vi "CRYGetPaneArea.vi"(11 "vi reference":refnum<vi>) -> (3 "Content Area Rect":T1)   [LabVIEW 2013]
uses:
  <vilib>/Utility/miscctls.llb/LVRectTypeDef.ctl
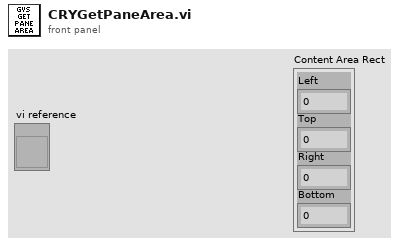
[diagram p1: front panel]
types:
  T1 = typedef "LVRectTypeDef.ctl" = cluster{"Left":i16, "Top":i16, "Right":i16, "Bottom":i16}
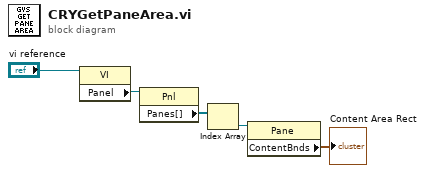
[diagram p0: block diagram]
diagram:
  n1 = property class="VI"(reference="vi reference") -> ("Panel"=w5:refnum<vi>)  [unwired: 1 in, 2 out]
  n2 = property class="Pnl"(reference=w5) -> ("Panes[]"=w4:refnum<vi>[])  [unwired: 1 in, 2 out]
  n3 = Index Array(array=w4) -> (element=w3:refnum<vi>)  [unwired: 1 in]
  n4 = property class="Pane"(reference=w3) -> ("ContentBnds"=→"Content Area Rect":T1)  [unwired: 1 in, 2 out]
